vi "Spd_Matrix.vi"(8 "error in (no error)":errorcluster caption="entrée d'erreur (pas d'erreur)", 11 "make_spd_matrix":cluster{"n_dim":u32, "random_state":i32}={"n_dim"=1, "random_state"=-1} {"random_state" min=-1; "n_dim" min=1}) -> (0 "error out":errorcluster, 3 "Data":T1)   [LabVIEW 2020]
doc: "Generate a random symmetric, positive-definite matrix.\n\n\nParameters : \n\n- n_dim : int\nThe matrix dimension.\n\n- random_state : int, RandomState instance, default=None=-1\nDetermines random number generation for dataset creation. Pass an int for reproducible output across multiple function calls. See Glossary.\n\nReturns : \n\n- X : array of shape [n_dim, n_dim]\nThe random symmetric, positive-definite matrix."
uses:
  Spd_Matrix.lvclass
panel:
  out "Spd_Matrix.lvclass":refnum<class "Spd_Matrix.lvclass">
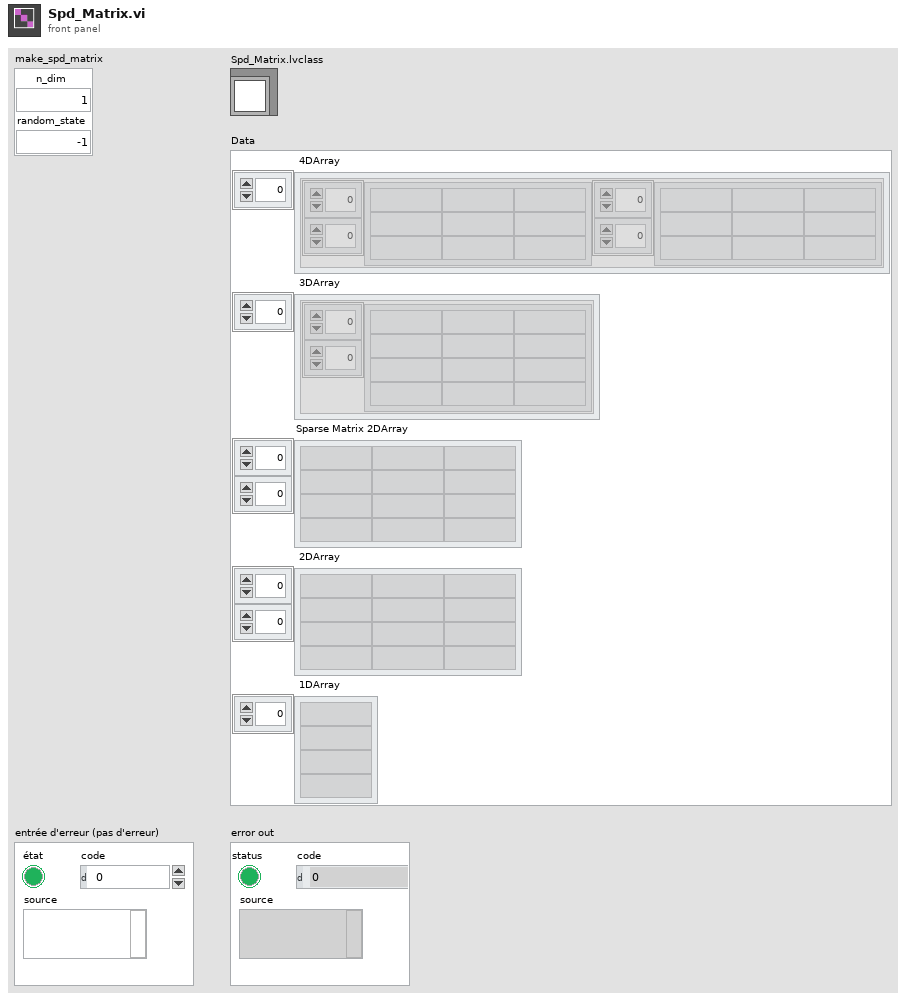
[diagram p1: front panel]
types:
  T1 = cluster{" 4DArray":cluster{"1":string[][], "2":string[][]}[], " 3DArray":cluster{"Tableau":string[][]}[], "Sparse Matrix 2DArray":string[][], " 2DArray":string[][], " 1DArray":string[]}
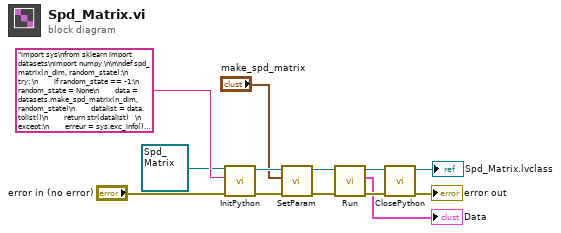
[diagram p0: block diagram]
diagram:
  n1 = call-dynamic "InitPython.vi"("error in (no error)"="error in (no error)", "Python Instruction"="import sys\nfrom sklearn import datasets\nimport numpy \n\n\ndef spd_matrix(n_dim, random_state):\n    try: \n        if random_state == -1:\n            random_state = None\n        data = datasets.make_spd_matrix(n_dim, random_state)\n        datalist = data.tolist()\n        return str(datalist)   \n    except:\n        erreur = sys.exc_info()\n        typerr = u\"%s\" % (erreur[0])\n        typerr = typerr[typerr.find(\"'\")+1:typerr.rfind(\"'\")]\n        msgerr = u\"%s\" % (erreur[1])\n        message = str('/!\\\\ {0} : {1}'. format(typerr,msgerr))\n        return message", "Scikit-learn en entrée"=refnum<class "Spd_Matrix.lvclass"> refnum ("Spd_Matrix.lvclass")) -> ("error out"=w9:errorcluster, "Scikit-learn en sortie"=w10:refnum<class "Spd_Matrix.lvclass">)  [unwired: 7 in]
  n2 = call-dynamic "SetParam.vi"("error in (no error)"=w9, "make_spd_matrix"="make_spd_matrix", "Spd_Matrix.lvclass"=w10) -> ("error out"=w6:errorcluster, "Spd_Matrix.lvclass"=w7:refnum<class "Spd_Matrix.lvclass">)  [unwired: 7 in]
  n3 = call-dynamic "Run.vi"("error in (no error)"=w6, "Spd_Matrix.lvclass"=w7) -> ("error out"=w4:errorcluster, "Data"=→"Data":T1, "Spd_Matrix.lvclass"=w5:refnum<class "Spd_Matrix.lvclass">)  [unwired: 7 in]
  n4 = call-dynamic "ClosePython.vi"("error in (no error)"=w4, "Scikit-learn en entrée"=w5) -> ("error out"=→"error out":errorcluster, "Scikit-learn en sortie"=→"Spd_Matrix.lvclass":refnum<class "Spd_Matrix.lvclass">)  [unwired: 8 in]
